vi "ComparationCOELBA.vi"() -> ()   [LabVIEW 2017]
uses:
  MainFGV/Settings/Advanced/AdvancedConfig.ctl
  Processing/results_data.ctl
  Post_processing/GraphMean/data_mean_plot.ctl
  Post_processing/GraphMean/plot_props.ctl
  Post_processing/GraphMean/axis_props.ctl
  <vilib>/Heliosphere Research LLC/Advanced Plotting Toolkit/api_core/NewPlotScales.ctl
  <vilib>/Analysis/NI_AALPro.lvlib
  <vilib>/Heliosphere Research LLC/Advanced Plotting Toolkit/Advanced Plotting Toolkit.lvlib
panel:
  in  "Ensaios":path[](array[path])
  in  "channel":i32=1 caption="Canal" min=1 max=4
  in  "stop":bool
  in  "log":bool
  in  "alpha":dbl=0.3 caption="Alpha" format="%#_6f"
  in  "maxFreq":dbl=72.0 caption="Frequência máxima" format="%#_g Hz"
  in  "minFreq":dbl=30.0 caption="Frequência mínima" format="%#_g Hz"
  in  "lowPass":dbl=1000.0 caption="Passa baixa" format="%#_g Hz"
  in  "highPass":dbl=1.0 caption="Passa alta" format="%#_g Hz"
  in  "Filtro":T1(ring)=enum."Passa banda"
  in  "cutoff":dbl=-6.0 caption="Cutoff amplitude [dB]" format="%#_g dB"
  in  "delete":bool
  in  "ok":bool
  in  "validate":bool
  in  "tab":enum32{"Batida individual", "Todas", "Media"}(tab)
  out "inert":waveform(dbl)[](graph) caption="Inertância"
  out "hammerSpec":waveform(dbl)(graph) caption="Martelo - Espectro"
  out "acelTime":waveform(dbl)[](graph) caption="Acelerômetros - Sinal no tempo"
  out "hammerTime":waveform(dbl)(graph) caption="Martelo - Sinal no tempo"
  out "meanInert":picture
  out "Picos":cluster{"freqs":dbl[], "Array":dbl[]}[](graph) caption="XY Graph"
  # "Análise modal\n\nAquisição\n\nLink do repositório: https://github.com/LeonardoSirino/ModalAnalysis"
  # "Leonardo Sirino\nSistemas Mecânicos \nT + 55 (41) 3361-6152 | C + 55 (41) 99679-007\nleonardo.sirino@lactec.org.br | www.lactec.org.br"
  # "Configurações para\napresentação"
  # "Configurações para\nprocessamento"
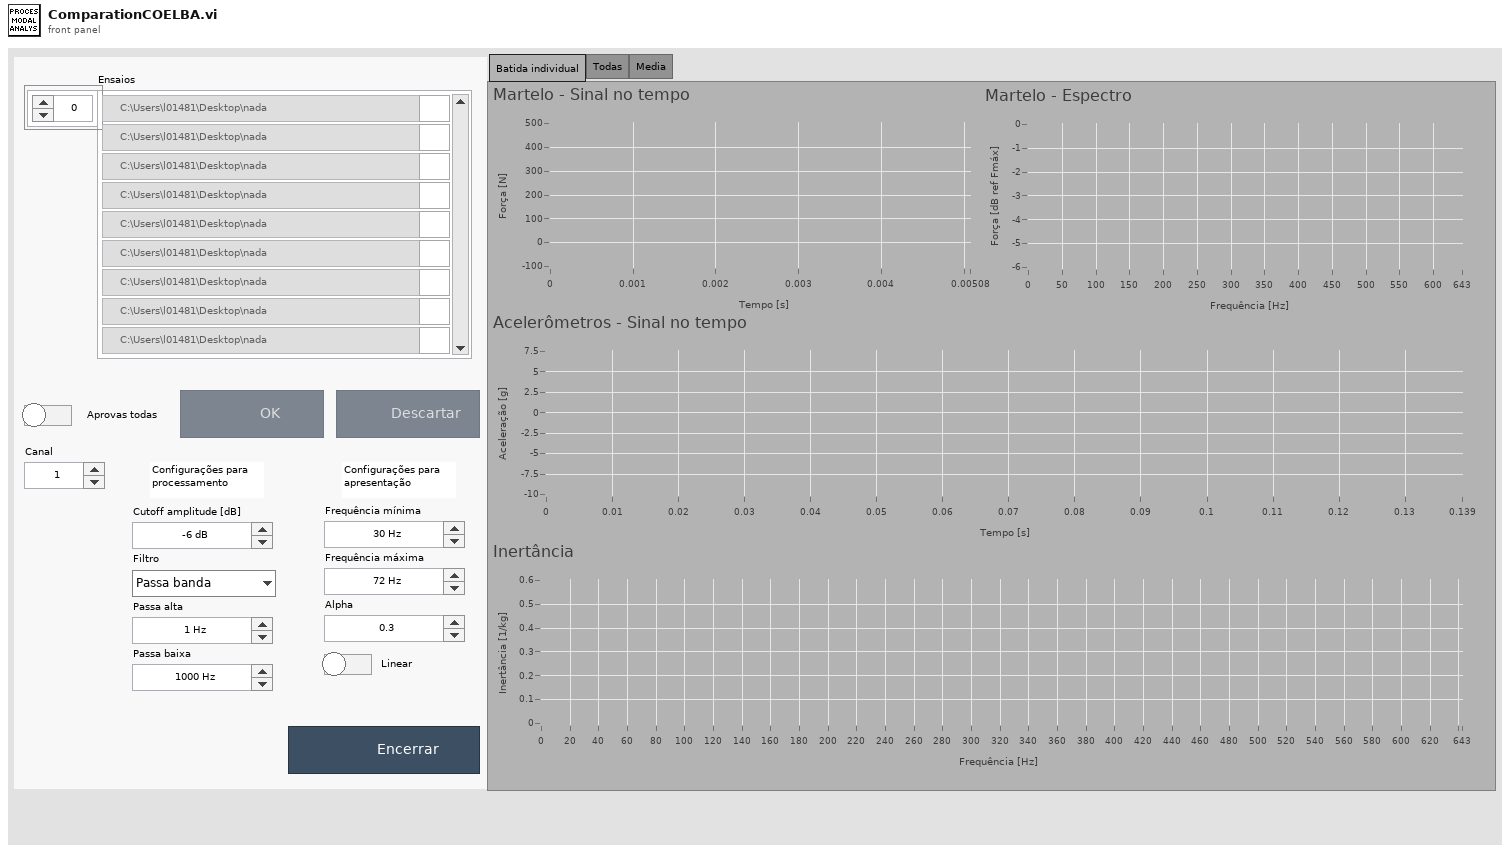
[diagram p1: front panel]
types:
  T1 = enum16{"Desativado", "Passa banda", "Passa alta", "Passa baixa"}
  T2 = enum8{"Enabled", "Disabled", "Disabled and Grayed Out"}
  T3 = typedef "AdvancedConfig.ctl" = cluster{"rate":dbl, "duration":dbl, "thr":dbl, "preTrigger":dbl, "cutoff":dbl, "Filtro":enum16{"Desativado", "Passa banda", "Passa alta", "Passa baixa"}, "highPass":dbl, "lowPass":dbl, "updateTime":dbl}
  T4 = typedef "results_data.ctl" = cluster{"config":T3, "hammer":waveform(dbl), "acelerometers":waveform(dbl)[], "hammerIndex":i32}
  T5 = cluster{"seconds since 1Jan1904":timestamp, "data_out":T4}
  T6 = typedef "data_mean_plot.ctl" = cluster{"array":dbl[], "dx":dbl, "x0":dbl}
  T7 = cluster{"seconds since 1Jan1904":timestamp, "data_out":T4}[]
  T8 = typedef "Advanced Plotting Toolkit.lvlib/NewPlotScales.ctl" = enum16{"Default", "Linear", "Log", "Symlog"}
  T9 = typedef "plot_props.ctl" = cluster{"x_axis":T10, "y_axis":T10, "y multiplier":dbl, "alpha":dbl, "base_tag":string, "itens_base_name":string, "graph_title":string, "plot_names":string[], "plot_all":bool}
  T10 = typedef "axis_props.ctl" = cluster{"min":dbl, "max":dbl, "label":string, "scale":T8}
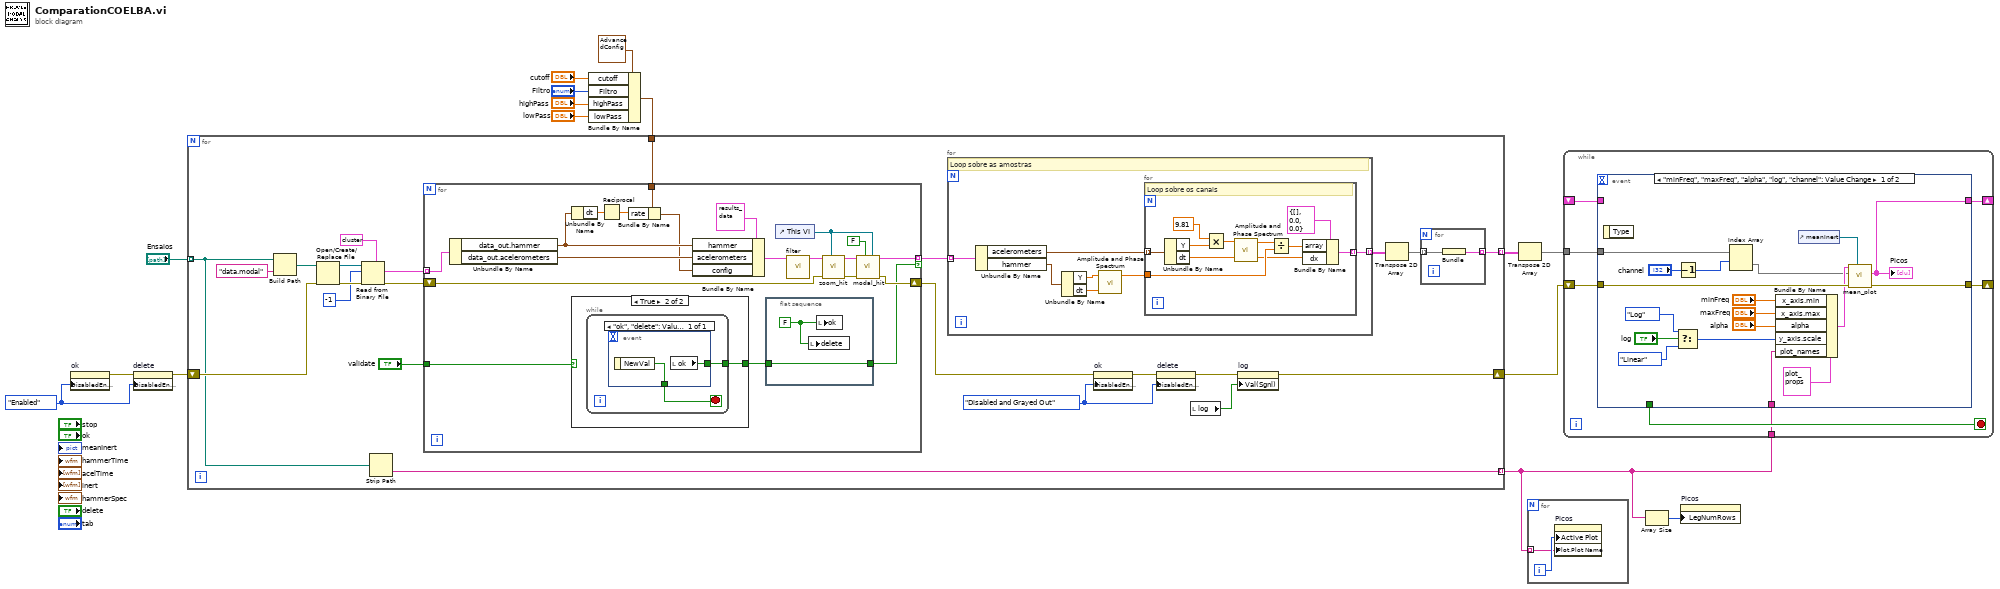
[diagram p0: block diagram]
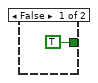
[diagram p2: hidden frame]
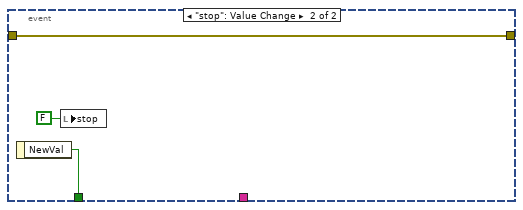
[diagram p3: hidden frame]
diagram:
  w8 = T2."Enabled" ("Disabled")
  n1 = property on="ok" class="Bool (strict)"("DisabledEnum"=w8) -> (error out=w7:errorcluster)  [unwired: 2 in, 1 out]
  n2 = property on="delete" class="Bool (strict)"(error in=w7, "DisabledEnum"=w8) -> (error out=w6:errorcluster)  [unwired: 1 in, 1 out]
  n3 = Bundle By Name(cluster=T3 {"rate"=1652.0, "duration"=1.0, "thr"=10.0, "preTrigger"=100.0, "cutoff"=-6.0, "Filtro"=enum."Passa banda", "highPass"=1.0, "lowPass"=1000.0, "updateTime"=50.0} ("config"), "cutoff"="cutoff", "Filtro"="Filtro", "highPass"="highPass", "lowPass"="lowPass") -> (w10:T3)
  n4 = for {
    tunnel: w10 -> [w31]
    tunnel: [w23] -> w4 mode=indexing
    shift-right: [w24] -> w9
    shift-left: w6 -> [w18]
    tunnel: "Ensaios" -> [w17] mode=indexing
    tunnel: [w16] -> w2 mode=indexing
    w20 = T2."Disabled and Grayed Out" ("Disabled")
    n5 = Build Path(base path=w17, name or relative path="data.modal") -> (appended path=w37:path)
    n6 = Open/Create/Replace File(file path (use dialog)=w37, error in=w18) -> (refnum out=w36:refnum<file>, error out=w34:errorcluster)  [unwired: 4 in, 1 out]
    n7 = Read from Binary File(5:T5 {"seconds since 1Jan1904"=timestamp(0 s since 1904-01-01), "data_out"={"config"={"rate"=0.0, "duration"=0.0, "thr"=0.0, "preTrigger"=0.0, "cutoff"=0.0, "Filtro"=enum."Desativado", "highPass"=0.0, "lowPass"=0.0, "updateTime"=0.0}, "hammer"={"t0"=timestamp(0 s since 1904-01-01), "dt"=1.0, "Y"=[]}, "acelerometers"=[], "hammerIndex"=0}} ("output cluster"), 8:w34, 10:-1 ("count (1)"), 11:w36) -> (0:w30:errorcluster, 2:w32:T7)  [unwired: 2 in, 2 out]
    n8 = Strip Path(path=w17) -> (name=w16:string)  [unwired: 1 out]
    n9 = for {
      tunnel: w32 -> [w78] mode=indexing
      tunnel: w31 -> [w68]
      shift-right: [w63] -> w22
      shift-left: w30 -> [w64]
      tunnel: [w61] -> w28 mode=indexing if=w60
      tunnel: "validate" -> [w59]
      n10 = Unbundle By Name(w78) -> ("data_out.hammer"=w69:waveform(dbl), "data_out.acelerometers"=w73:waveform(dbl)[])
      n11 = case shown="True" w59 {
        tunnel: [TRUE ("ok") w82] -> w62
        frame False {
        }
        frame True {
          n12 = while {
            tunnel: [w84] -> w82
            stop <- w83 stop-if-true
            n13 = event shown="[0] \"ok\", \"delete\": Value Change" {
              selector: _ -> [_]
              dyn-events: _ -> [_]
              timeout: _ -> [_]
              tunnel: [w85] -> w84
              tunnel: [w86] -> w83
              event "ok", "delete": Value Change {
                n14 = event-data() -> ("NewVal"=w86:bool)  [unwired: 1 in]
                n15 = local read "ok"() -> (w85:bool)
              }
            }
          }
        }
      }
      n16 = Unbundle By Name(w69) -> ("dt"=w67:dbl)
      n17 = Reciprocal(x=w67) -> (1/x=w66:dbl)
      n18 = Bundle By Name(cluster=w68, "rate"=w66) -> (w65:T3)
      n19 = Bundle By Name(cluster=T4 {"config"={"rate"=0.0, "duration"=0.0, "thr"=0.0, "preTrigger"=0.0, "cutoff"=0.0, "Filtro"=enum."Desativado", "highPass"=0.0, "lowPass"=0.0, "updateTime"=0.0}, "hammer"={"t0"=timestamp(0 s since 1904-01-01), "dt"=1.0, "Y"=[]}, "acelerometers"=[], "hammerIndex"=0} ("data_in"), "hammer"=w69, "acelerometers"=w73, "config"=w65) -> (w72:T4)
      n20 = flat-sequence {
        tunnel: w62 -> [w80]
        tunnel: [w80] -> w60
        frame #0 {
          w79 = FALSE ("ok")
          n21 = local write "delete"(w79) -> ()
          n22 = local write "ok"(w79) -> ()
        }
      }
      n23 = control-ref of="This VI"() -> (w71:refnum<vi>)
      n24 = call "filter.vi"("data_in"=w72) -> ("data_out"=w75:T4)  [unwired: 9 in, 1 out]
      n25 = call "zoom_hit.vi"("refVI"=w71, "error in"=w64, "data_in"=w75) -> ("error out"=w76:errorcluster, "data_out"=w77:T4)  [unwired: 7 in]
      n26 = call "modal_hit.vi"("refVI"=w71, "acquisition"=FALSE, "error in"=w76, "data_in"=w77) -> ("error out"=w63:errorcluster, "data_out"=w61:T4)  [unwired: 6 in]
    }
    n27 = for {
      tunnel: w28 -> [w47] mode=indexing
      tunnel: [w41] -> w27 mode=indexing
      # "Loop sobre as amostras"
      n28 = Unbundle By Name(w47) -> ("acelerometers"=w46:waveform(dbl)[], "hammer"=w43:waveform(dbl))
      n29 = Unbundle By Name(w43) -> ("Y"=w44:dbl[], "dt"=w45:dbl)
      n30 = call <vilib>:"Amplitude and Phase Spectrum.vi"("dt"=w45, "Signal (V)"=w44) -> ("Amp Spectrum Mag (Vrms)"=w42:dbl[])  [unwired: 1 in, 2 out]
      n31 = for {
        tunnel: w46 -> [w58] mode=indexing
        tunnel: w42 -> [w52]
        tunnel: [w48] -> w41 mode=indexing
        # "Loop sobre os canais"
        n32 = Unbundle By Name(w58) -> ("Y"=w57:dbl[], "dt"=w54:dbl)
        n33 = Multiply(x=9.81, y=w57) -> (x*y=w55:dbl[])
        n34 = call <vilib>:"Amplitude and Phase Spectrum.vi"("dt"=w54, "Signal (V)"=w55) -> ("df"=w49:dbl, "Amp Spectrum Mag (Vrms)"=w53:dbl[])  [unwired: 1 in, 1 out]
        n35 = Divide(x=w53, y=w52) -> (x/y=w50:dbl[])
        n36 = Bundle By Name(cluster=T6 {"array"=[], "dx"=0.0, "x0"=0.0} ("data_mean_plot"), "array"=w50, "dx"=w49) -> (w48:T6)
      }
    }
    n37 = property on="ok" class="Bool (strict)"(error in=w22, "DisabledEnum"=w20) -> (error out=w21:errorcluster)  [unwired: 1 in, 1 out]
    n38 = property on="delete" class="Bool (strict)"(error in=w21, "DisabledEnum"=w20) -> (error out=w19:errorcluster)  [unwired: 1 in, 1 out]
    n39 = local read "log"() -> (w25:bool)
    n40 = property on="log" class="Bool (strict)"(error in=w19, "Val(Sgnl)"=w25) -> (error out=w24:errorcluster)  [unwired: 1 in, 1 out]
    n41 = Transpose 2D Array(2D array=w27) -> (transposed array=w26:T6[][])
    n42 = for {
      tunnel: w26 -> [w40] mode=indexing
      tunnel: [w39] -> w23 mode=indexing
      n43 = Bundle(w40) -> (w39:cluster{T6[]})  [unwired: 1 in]
    }
  }
  n44 = Transpose 2D Array(2D array=w4) -> (transposed array=w3:cluster{T6[]}[][])
  n45 = for {
    tunnel: w2 -> [w87] mode=indexing
    i -> [w88]
    n46 = property on="Picos" class="XYGraph (strict)"("Active Plot"=w88, "Plot.Plot Name"=w87) -> ()  [unwired: 2 in, 2 out]
  }
  n47 = while {
    shift-right: [w94] -> _
    shift-left: _ -> [w95]
    shift-right: [w93] -> _
    shift-left: w9 -> [w92]
    tunnel: w3 -> [w90]
    tunnel: w2 -> [w89]
    stop <- w91 stop-if-true
    n48 = event shown="[0] \"minFreq\", \"maxFreq\", \"alpha\", \"log\", \"channel\": Value Change" {
      selector: _ -> [_ _]
      dyn-events: _ -> [_ _]
      timeout: _ -> [_ _]
      tunnel: w95 -> [_ _]
      tunnel: [w98 _] -> w94
      tunnel: [w102 w115] -> w93
      tunnel: w92 -> [w112 w115]
      tunnel: [_ w116] -> w91
      tunnel: w90 -> [w101 _]
      tunnel: w89 -> [w97 _]
      event "minFreq", "maxFreq", "alpha", "log", "channel": Value Change {
        n49 = event-data() -> ()  [unwired: 1 in, 1 out]
        n50 = Select(t=NewPlotScales."Log" ("y_axis.scale"), s="log", f=NewPlotScales."Linear" ("y_axis.scale")) -> (s? t:f=w111:T8)
        n51 = Decrement(x="channel") -> (x-1=w96:i32)
        n52 = Index Array(array=w101, index (row)=w96) -> (element=w100:cluster{T6[]}[])  [unwired: 1 in]
        n53 = Bundle By Name(cluster=T9 {"x_axis"={"min"=30.0, "max"=72.0, "label"="Frequência [Hz]", "scale"=enum."Default"}, "y_axis"={"min"=nan, "max"=nan, "label"="Inertância [1/kg]", "scale"=enum."Linear"}, "y multiplier"=1.0, "alpha"=0.5, "base_tag"="", "itens_base_name"="", "graph_title"="Inertância média", "plot_names"=[], "plot_all"=TRUE} ("plot_properties"), "x_axis.min"="minFreq", "x_axis.max"="maxFreq", "alpha"="alpha", "y_axis.scale"=w111, "plot_names"=w97) -> (w103:T9)
        n54 = control-ref of="meanInert"() -> (w113:refnum<vi>)
        n55 = call "mean_plot.vi"("ref_picture"=w113, "error in"=w112, "channels"=w100, "plot_properties"=w103) -> ("error out"=w102:errorcluster, "mean_curves"=w98:cluster{"freqs":dbl[], "Array":dbl[]}[])  [unwired: 5 in, 1 out]
        "Picos" <- w98
      }
      event "stop": Value Change {
        n56 = event-data() -> ("NewVal"=w116:bool)  [unwired: 1 in]
        n57 = local write "stop"(FALSE ("stop")) -> ()
      }
    }
  }
  n58 = Array Size(array=w2) -> (size(s)=w1:i32)
  n59 = property on="Picos" class="XYGraph (strict)"("LegNumRows"=w1) -> ()  [unwired: 2 in, 2 out]
